vi "Set Motor Direction.vi"(8 "error in (no error)":errorcluster, 9 "Direction":T1, 10 "Motor":u16, 11 "Grove I2C L298P Motor Drive in":refnum<class "Grove I2C L298P Motor Drive.lvclass">) -> (0 "error out":errorcluster, 3 "Grove I2C L298P Motor Drive out":refnum<class "Grove I2C L298P Motor Drive.lvclass">)   [LabVIEW 2020, in "CTI-Peripheral.lvlib" / "Grove I2C L298P Motor Drive.lvclass"]
uses:
  Grove I2C L298P Motor Drive.lvclass
  Base/Direction.ctl
  Grove I2C L298P Motor Drive.lvclass/Grove I2C L298P Motor Drive.ctl
  CTI/I2C Connection/I2C Connection.lvclass/I2C Connection.ctl
  CTI/Session/I2C Write Data.vi
  CTI/I2C Connection/I2C Connection.lvclass
  Base/Motor Controller.lvclass
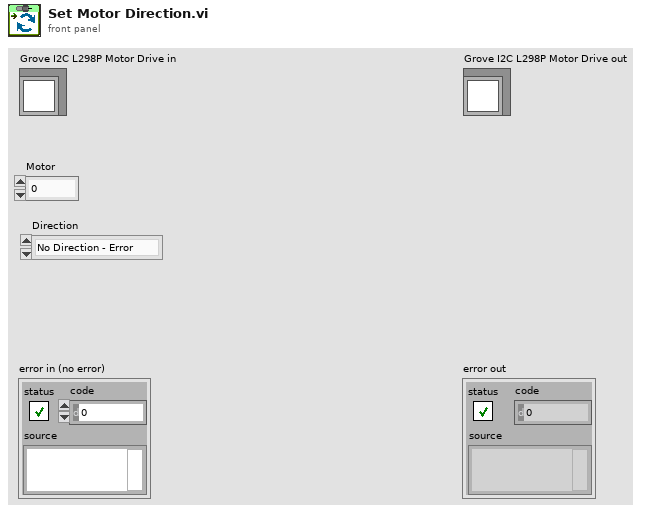
[diagram p1: front panel]
types:
  T1 = typedef "CTI-Peripheral.lvlib/Motor Controller.lvclass/Direction.ctl" = enum16{"No Direction - Error", "Clockwise (CW)", "Anti-Clockwise (ACW)"}
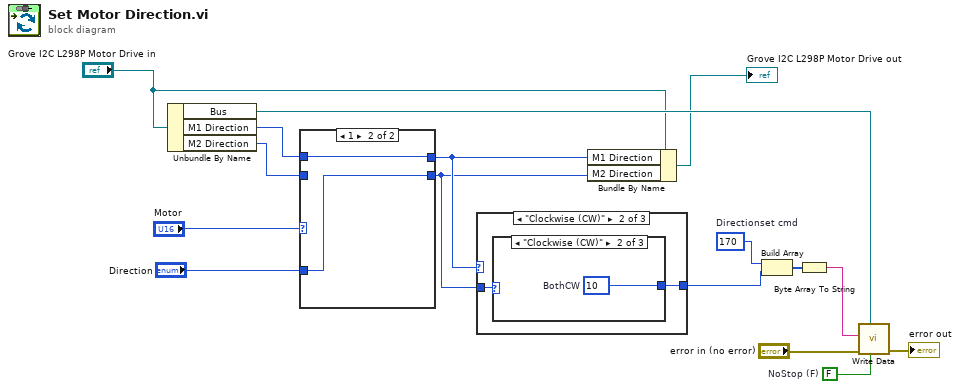
[diagram p0: block diagram]
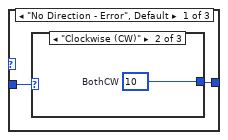
[diagram p2: hidden frame]
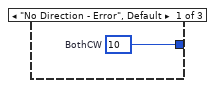
[diagram p3: hidden frame]
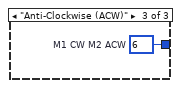
[diagram p4: hidden frame]
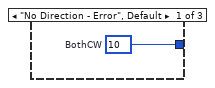
[diagram p5: hidden frame]
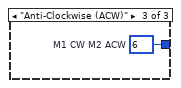
[diagram p6: hidden frame]
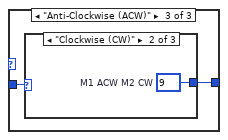
[diagram p7: hidden frame]
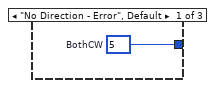
[diagram p8: hidden frame]
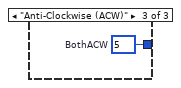
[diagram p9: hidden frame]
diagram:
  w13 = u8 170  # Directionset cmd
  w14 = FALSE  # NoStop (F)
  n1 = Unbundle By Name("Grove I2C L298P Motor Drive in") -> ("Bus"=w15:refnum<class "I2C Connection.lvclass">, "M1 Direction"=w5:T1, "M2 Direction"=w4:T1)
  n2 = case shown="1" "Motor" {
    tunnel: "Direction" -> [w17 w19]
    tunnel: w5 -> [_ w20]
    tunnel: w4 -> [w18 _]
    tunnel: [w18 w19] -> w2
    tunnel: [w17 w20] -> w3
    frame 0, Default {
    }
    frame 1 {
    }
  }
  n3 = case shown="\"Clockwise (CW)\"" w3 {
    tunnel: w2 -> [w22 w27 w32]
    tunnel: [w21 w26 w31] -> w1
    frame "No Direction - Error", Default {
      n4 = case shown="\"Clockwise (CW)\"" w22 {
        tunnel: [w23 w24 w25] -> w21
        frame "No Direction - Error", Default {
          w23 = u8 10  # BothCW
        }
        frame "Clockwise (CW)" {
          w24 = u8 10  # BothCW
        }
        frame "Anti-Clockwise (ACW)" {
          w25 = u8 6  # M1 CW M2 ACW
        }
      }
    }
    frame "Clockwise (CW)" {
      n5 = case shown="\"Clockwise (CW)\"" w27 {
        tunnel: [w28 w29 w30] -> w26
        frame "No Direction - Error", Default {
          w28 = u8 10  # BothCW
        }
        frame "Clockwise (CW)" {
          w29 = u8 10  # BothCW
        }
        frame "Anti-Clockwise (ACW)" {
          w30 = u8 6  # M1 CW M2 ACW
        }
      }
    }
    frame "Anti-Clockwise (ACW)" {
      n6 = case shown="\"Clockwise (CW)\"" w32 {
        tunnel: [w33 w34 w35] -> w31
        frame "No Direction - Error", Default {
          w33 = u8 5  # BothCW
        }
        frame "Clockwise (CW)" {
          w34 = u8 9  # M1 ACW M2 CW
        }
        frame "Anti-Clockwise (ACW)" {
          w35 = u8 5  # BothACW
        }
      }
    }
  }
  n7 = Bundle By Name(cluster="Grove I2C L298P Motor Drive in", "M1 Direction"=w3, "M2 Direction"=w2) -> (→"Grove I2C L298P Motor Drive out":refnum<class "Grove I2C L298P Motor Drive.lvclass">)
  n8 = Build Array(w13, w1) -> (w12:u8[])
  n9 = Byte Array To String(unsigned byte array=w12) -> (string=w10:string)
  n10 = call "Write Data.vi"("NoStop (F)"=w14, "I2C Connection"=w15, "error in (no error)"="error in (no error)", "Data"=w10) -> ("error out"=→"error out":errorcluster)  [unwired: 7 in]
